vi "Get Timing Grp.vi"(8 "error in (no error)":errorcluster, 10 "Timing Engine":T1=enum."Low Speed", 11 "Chassis Cfg":refnum<class "ChassisCfg.lvclass">) -> (0 "error out":errorcluster, 2 "Timing Groups":refnum<class "TimingGrp.lvclass">, 3 "Chassis Cfg":refnum<class "ChassisCfg.lvclass">)   [LabVIEW 2012, in "Configuration Grandmaster.lvlib" / "ChassisCfg.lvclass"]
uses:
  ChassisCfg.lvclass
  Common/Controls/TE_Designator.ctl
  Class Timing Group/TimingGrp.lvclass
  ChassisCfg.lvclass/ChassisCfg.ctl
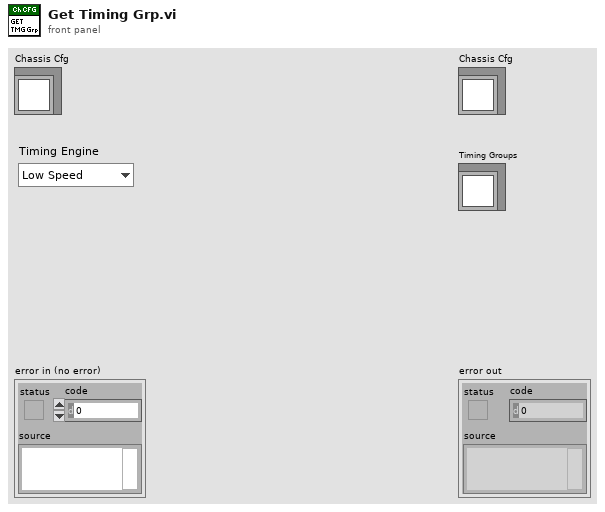
[diagram p1: front panel]
types:
  T1 = typedef "TE_Designator.ctl" = enum16{"High Speed", "Low Speed"}
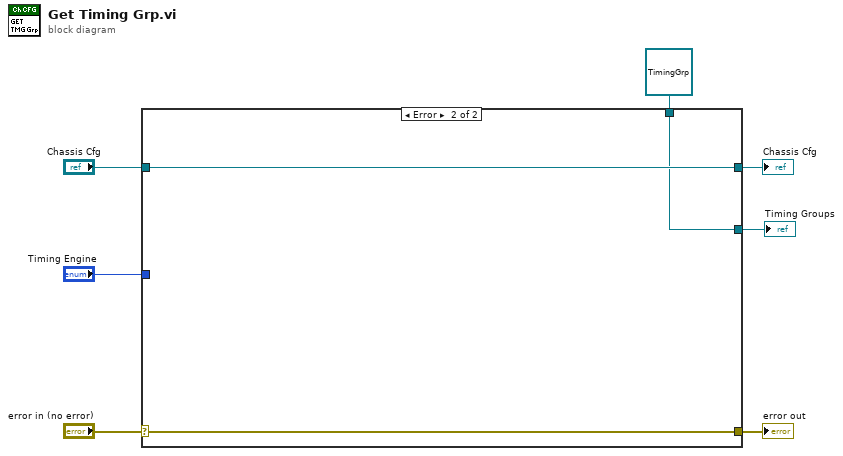
[diagram p0: block diagram]
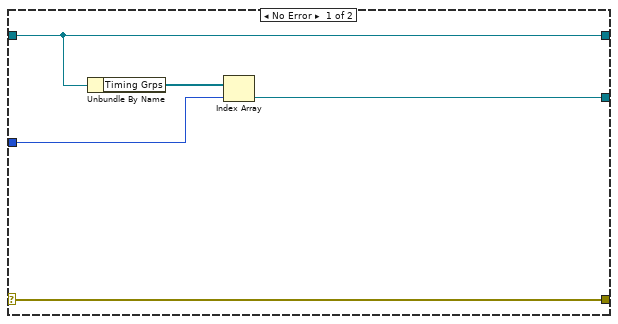
[diagram p2: hidden frame]
diagram:
  n1 = case shown="Error" "error in (no error)" {
    selector: "error in (no error)" -> [w12 w15]
    tunnel: [w12 w15] -> w6
    tunnel: [w11 w14] -> w4
    tunnel: "Chassis Cfg" -> [w11 w14]
    tunnel: "Timing Engine" -> [w9 _]
    tunnel: [w8 w13] -> w2
    tunnel: refnum<class "TimingGrp.lvclass"> refnum ("Timing Grp") -> [_ w13]
    frame No Error {
      n2 = Unbundle By Name(w11) -> ("Timing Grps"=w10:refnum<class "TimingGrp.lvclass">[])
      n3 = Index Array(array=w10, index=w9) -> (element=w8:refnum<class "TimingGrp.lvclass">)
    }
    frame Error {
    }
  }
  "error out" <- w6
  "Chassis Cfg" <- w4
  "Timing Groups" <- w2
